vi "Downsample_Filter_Test_32bit.vi"() -> ()   [LabVIEW 2025]
uses:
  <vilib>/measure/maspectr.llb/Power Spectrum and PSD Export Mode.ctl
  <vilib>/measure/maspectr.llb/FFT Power Spectrum and PSD for 1 Chan.vi
  <vilib>/measure/NI_MAPro.lvlib
panel:
  in  "Constant signal":bool
  out "original size":i32
  out "filtered size":i32
  out "Output valid":i16[](graph)
  out "filtered numeric":dbl[](array[numeric])
  out "Filtered signal":dbl[](graph)
  out "Power spectrum in":cluster{"f0":dbl, "df":dbl, "magnitude":dbl[]}(graph)
  out "Power spectrum out":cluster{"f0":dbl, "df":dbl, "magnitude":dbl[]}[](graph)
  out "Input signal":dbl[](graph)
  out "# of Iterations":i32
  out "# of samples":i32
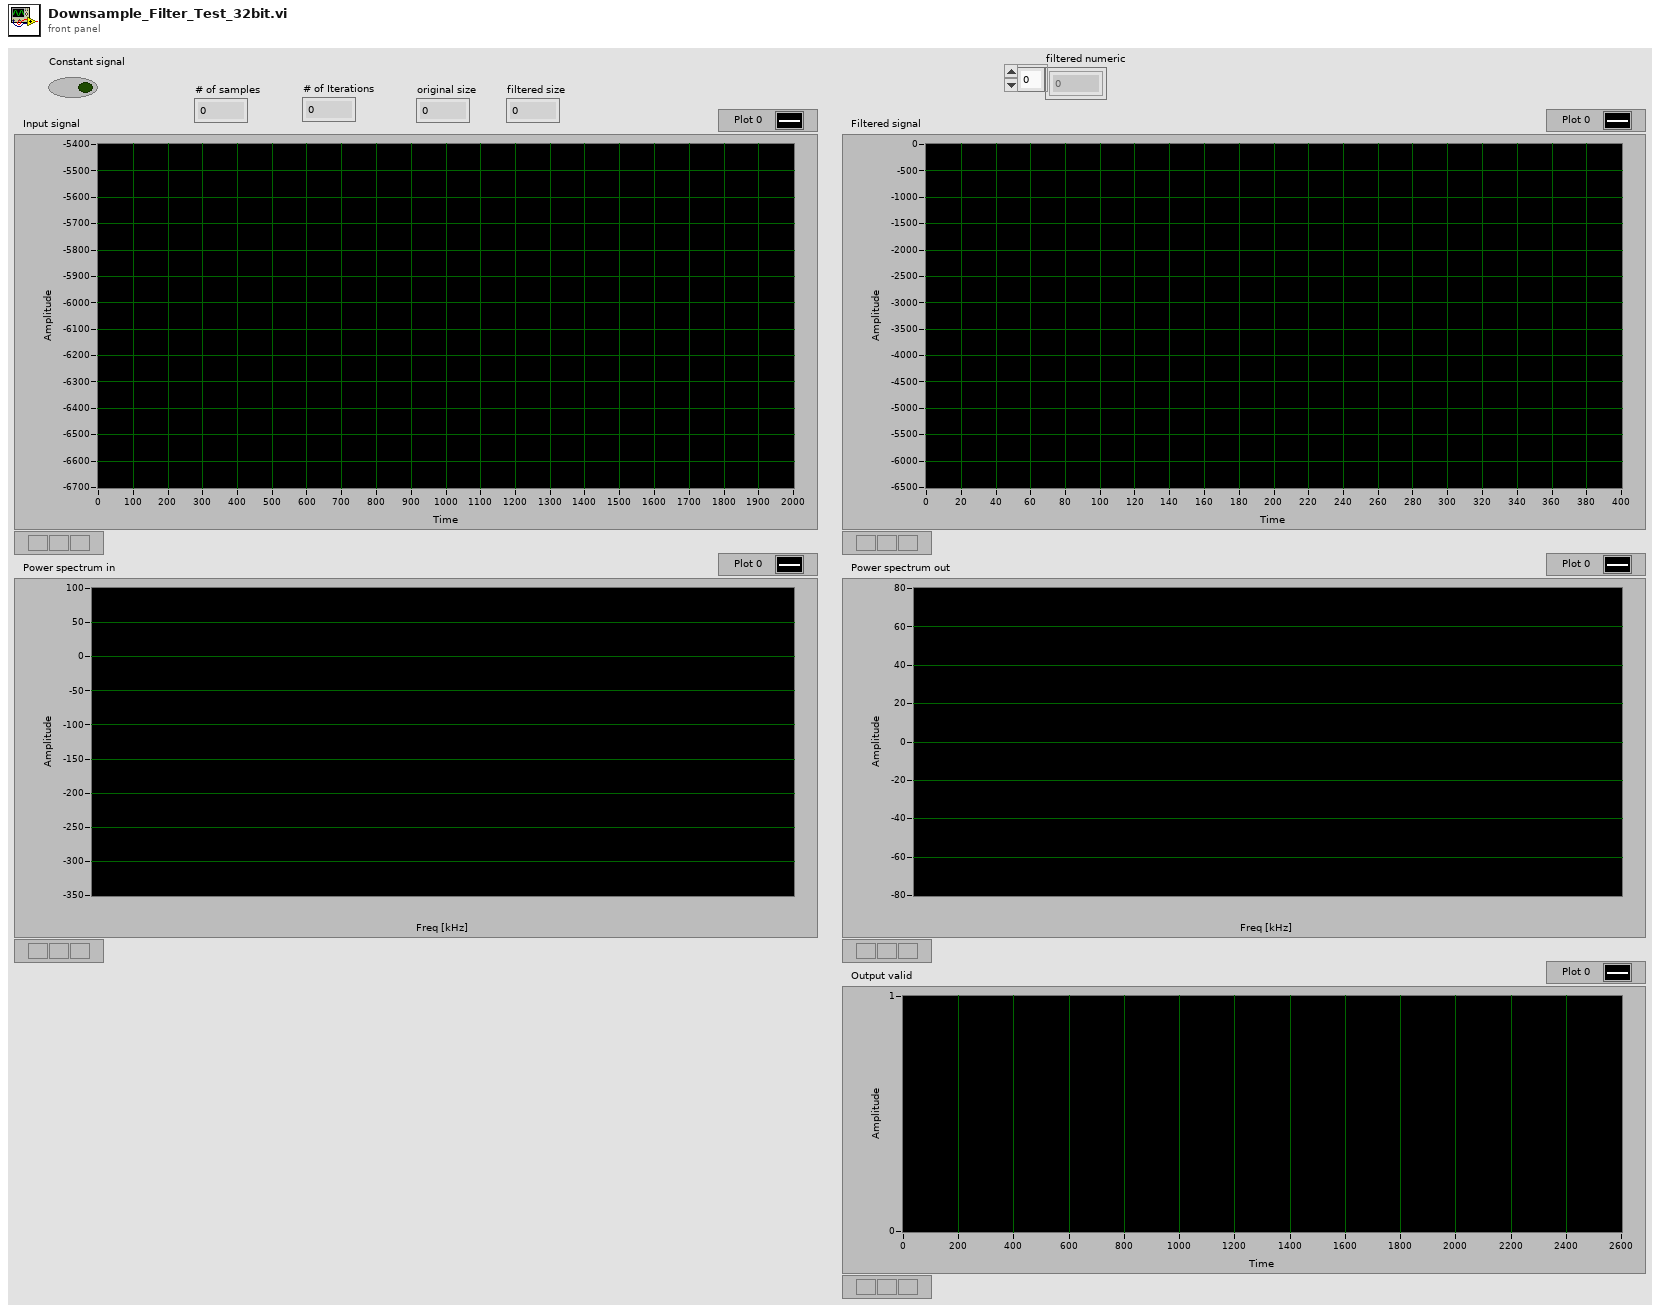
[diagram p1: front panel]
types:
  T1 = typedef "NI_MAPro.lvlib/Power Spectrum and PSD Export Mode.ctl" = u16
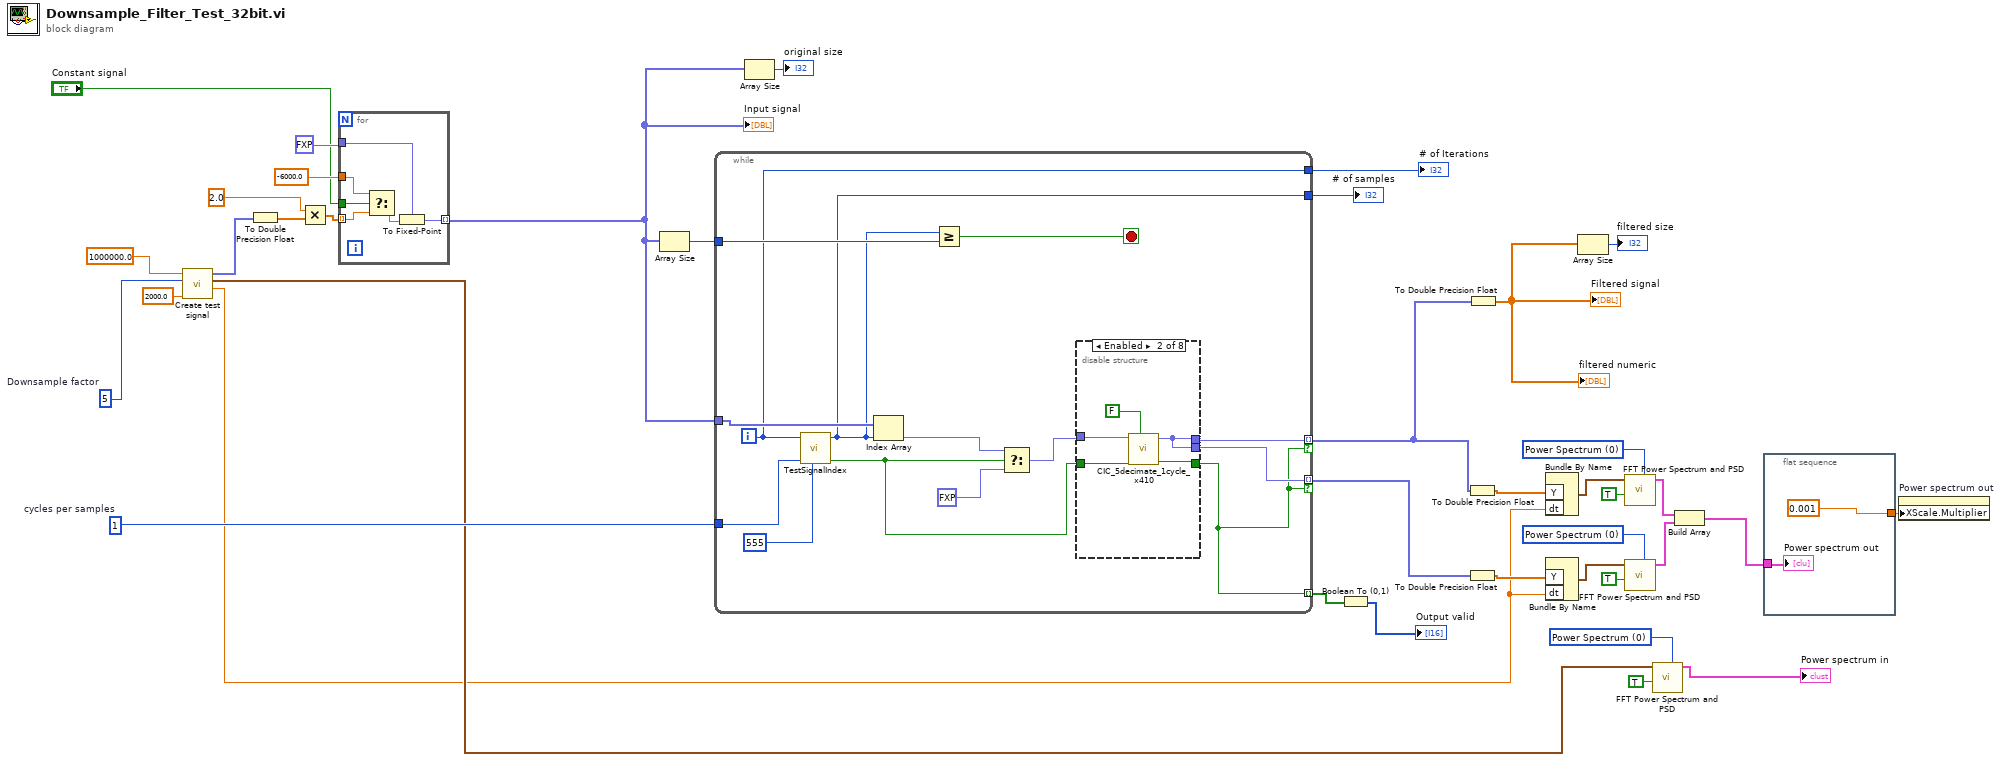
[diagram p0: block diagram]
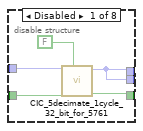
[diagram p2: hidden frame]
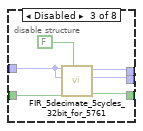
[diagram p3: hidden frame]
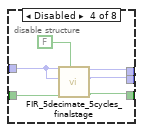
[diagram p4: hidden frame]
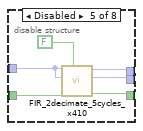
[diagram p5: hidden frame]
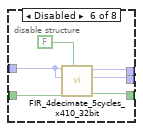
[diagram p6: hidden frame]
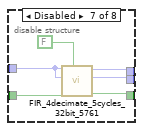
[diagram p7: hidden frame]
diagram:
  w22 = T1 0 items=["Power Spectrum", "Power Spectral Density"] ("export mode")
  w27 = 5  # Downsample factor
  w31 = 1  # cycles per samples
  w33 = T1 0 items=["Power Spectrum", "Power Spectral Density"] ("export mode")
  w37 = T1 0 items=["Power Spectrum", "Power Spectral Density"] ("export mode")
  n1 = call "Create test signal.vi"("Number of samples"=2000.0, "Downsample factor"=w27, "Sample rate"=1000000.0) -> ("dt"=w16:dbl, "signal out"=w29:waveform(dbl), "Y"=w8:fxp<+/-,16,14>[])  [unwired: 6 in]
  n2 = To Double Precision Float(number=w8) -> (double precision float=w4:dbl[])
  n3 = Multiply(x=2.0 ("fixed-point type"), y=w4) -> (x*y=w2:dbl[])
  n4 = for {
    tunnel: w2 -> [w42] mode=indexing
    tunnel: fxp<+/-,32,14> 0.0 ("Q in") -> [w45]
    tunnel: [w44] -> w6 mode=indexing
    tunnel: -6000.0 ("fixed-point type") -> [w43]
    tunnel: "Constant signal" -> [w40]
    n5 = Select(t=w43, s=w40, f=w42) -> (s? t:f=w41:dbl)
    n6 = To Fixed-Point(fixed-point type=w45, number=w41) -> (fixed-point=w44:fxp<+/-,32,14>)
  }
  "Input signal" <- w6
  n7 = Array Size(array=w6) -> (size(s)=w39:i32)
  n8 = while {
    tunnel: w6 -> [w59]
    tunnel: [w56] -> w19 mode=indexing if=w48
    tunnel: w39 -> [w57]
    tunnel: w31 -> [w55]
    tunnel: [w48] -> w30 mode=indexing
    tunnel: [w49] -> w18 mode=indexing if=w48
    tunnel: [w47] -> w11
    tunnel: [w46] -> w10
    i -> [w46]
    stop <- w58 stop-if-true
    n9 = call "TestSignalIndex.vi"("initial delay"=555, "cycles per sample"=w55, "index"=w46) -> ("valid out"=w50:bool, "array index"=w47:i32)  [unwired: 7 in]
    n10 = Index Array(array=w59, index=w47) -> (element=w54:fxp<+/-,32,14>)
    n11 = Greater Or Equal?(x=w47, y=w57) -> (x >= y?=w58:bool)
    n12 = Select(t=w54, s=w50, f=fxp<+/-,32,14> 0.0) -> (s? t:f=w53:fxp<+/-,32,14>)
    n13 = disable-structure shown="Enabled" {
      disable-tunnel: [w60 w65 w75 w77 w87 w93 w99 _] -> w56
      disable-tunnel: w53 -> [w64 w69 w74 w81 w86 w92 w98 _]
      disable-tunnel: w50 -> [w63 w68 w73 w79 w85 w91 w97 _]
      disable-tunnel: [w60 w65 w72 w78 w84 w90 w96 _] -> w49
      disable-tunnel: [w62 w67 w71 w76 w83 w89 w95 _] -> w48
      frame Disabled {
        n14 = call "CIC_5decimate_1cycle_32_bit_for_5761.vi"("reset"=FALSE, "valid in"=w63, "Data in"=w64) -> ("valid out"=w62:bool, "Data out"=w60:fxp<+/-,32,14>)  [unwired: 7 in]
      }
      frame Enabled {
        n15 = call "CIC_5decimate_1cycle_x410.vi"("reset"=FALSE, "valid in"=w68, "Data in"=w69) -> ("valid out"=w67:bool, "Data out"=w65:fxp<+/-,32,14>)  [unwired: 7 in]
      }
      frame Disabled {
        n16 = call "FIR_5decimate_5cycles_32bit_for_5761.vi"("reset"=FALSE, "valid in"=w73, "Q in"=w74, "I in"=w74) -> ("valid out"=w71:bool, "Q out"=w72:fxp<+/-,32,14>, "I out"=w75:fxp<+/-,32,14>)  [unwired: 4 in, 1 out]
      }
      frame Disabled {
        n17 = call "FIR_5decimate_5cycles_finalstage.vi"("reset"=FALSE, "valid in"=w79, "Q in"=w81, "I in"=w81) -> ("valid out"=w76:bool, "Q out"=w78:fxp<+/-,32,14>, "I out"=w77:fxp<+/-,32,14>)  [unwired: 4 in, 1 out]
      }
      frame Disabled {
        n18 = call "FIR_2decimate_5cycles_x410.vi"("reset"=FALSE, "valid in"=w85, "Q in"=w86, "I in"=w86) -> ("valid out"=w83:bool, "Q out"=w84:fxp<+/-,32,14>, "I out"=w87:fxp<+/-,32,14>)  [unwired: 4 in, 1 out]
      }
      frame Disabled {
        n19 = call "FIR_4decimate_5cycles_x410_32bit.vi"("reset"=FALSE, "valid in"=w91, "Q in"=w92, "I in"=w92) -> ("valid out"=w89:bool, "Q out"=w90:fxp<+/-,32,14>, "I out"=w93:fxp<+/-,32,14>)  [unwired: 4 in, 1 out]
      }
      frame Disabled {
        n20 = call "FIR_4decimate_5cycles_32bit_5761.vi"("reset"=FALSE, "valid in"=w97, "Q in"=w98, "I in"=w98) -> ("valid out"=w95:bool, "Q out"=w96:fxp<+/-,32,14>, "I out"=w99:fxp<+/-,32,14>)  [unwired: 4 in, 1 out]
      }
      frame Disabled {
      }
    }
  }
  "# of samples" <- w11
  "# of Iterations" <- w10
  n21 = Array Size(array=w6) -> (size(s)=→"original size":i32)
  n22 = Boolean To (0,1)(Boolean=w30) -> (0, 1=→"Output valid":i16[])
  n23 = To Double Precision Float(number=w19) -> (double precision float=w25:dbl[])
  n24 = To Double Precision Float(number=w18) -> (double precision float=w35:dbl[])
  n25 = To Double Precision Float(number=w19) -> (double precision float=w14:dbl[])
  "Filtered signal" <- w14
  "filtered numeric" <- w14
  n26 = Bundle By Name("Y"=w25, "dt"=w16) -> (w23:waveform(dbl))  [unwired: 1 in]
  n27 = Bundle By Name("Y"=w35, "dt"=w16) -> (w38:waveform(dbl))  [unwired: 1 in]
  n28 = Array Size(array=w14) -> (size(s)=→"filtered size":i32)
  n29 = call-poly <vilib>:"FFT Power Spectrum and PSD.vi"("export mode"=w22, "dB On (F)"=TRUE, "time signal"=w23) -> ("Power Spectrum / PSD"=w20:cluster{"f0":dbl, "df":dbl, "magnitude":dbl[]})  [unwired: 5 in, 3 out]
  n30 = call-poly <vilib>:"FFT Power Spectrum and PSD.vi"("export mode"=w37, "dB On (F)"=TRUE, "time signal"=w38) -> ("Power Spectrum / PSD"=w21:cluster{"f0":dbl, "df":dbl, "magnitude":dbl[]})  [unwired: 5 in, 3 out]
  n31 = call-poly <vilib>:"FFT Power Spectrum and PSD.vi"("export mode"=w33, "dB On (F)"=TRUE, "time signal"=w29) -> ("Power Spectrum / PSD"=→"Power spectrum in":cluster{"f0":dbl, "df":dbl, "magnitude":dbl[]})  [unwired: 5 in, 3 out]
  n32 = Build Array(w20, w21) -> (w17:cluster{"f0":dbl, "df":dbl, "magnitude":dbl[]}[])
  n33 = flat-sequence {
    tunnel: w17 -> [w101]
    tunnel: [0.001 ("X Scale.Offset and Multiplier:Multiplier")] -> w15
    frame #0 {
      "Power spectrum out" <- w101
    }
  }
  n34 = property on="Power spectrum out" class="WFGraph (strict)"("XScale.Multiplier"=w15) -> ()  [unwired: 2 in, 2 out]
